vi "PH_Stepmotor_BaseClass.ProcPeriodic.vi"(0 "i ref in":refnum<vi>, 3 "ms timeout":i32=100, 5 "error in":errorcluster) -> (14 "i ref out":refnum<vi>, 17 "time out?":bool, 19 "error out":errorcluster)   [LabVIEW 2014, in "PH_Stepmotor_BaseClass.lvlib"]
doc: "This method serves to periodically do things like reading values from the HW. Methods that should be executed periodically should be called from THIS methode. Add code here."
uses:
  PH_Stepmotor_BaseClass.lvlib
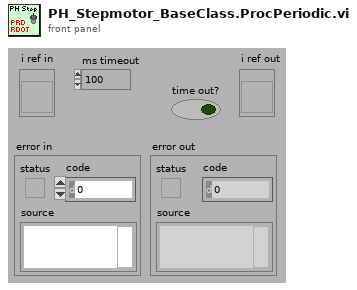
[diagram p1: front panel]
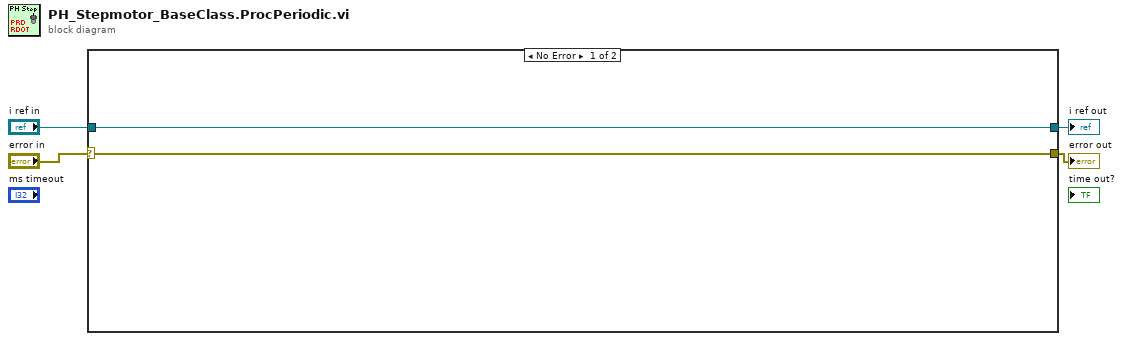
[diagram p0: block diagram]
diagram:
  n1 = case shown="No Error" "error in" {
    selector: "error in" -> [w5 w7]
    tunnel: [w6 w8] -> w4
    tunnel: "i ref in" -> [w6 w8]
    tunnel: [w5 w7] -> w1
    frame No Error {
    }
    frame Error {
    }
  }
  "error out" <- w1
  "i ref out" <- w4
